vi "Test Report Contain Failiing TestCase Name.vi"(8 "error in (no error)":errorcluster, 11 "XML Report Test in":refnum<class "XML Report Test.lvclass">) -> (0 "error out":errorcluster, 3 "XML Report Test out":refnum<class "XML Report Test.lvclass">)   [LabVIEW 2020, in "XML Report Test.lvclass"]
uses:
  XML Report Test.lvclass
  source/Plugins/XML Report/XML Report.lvclass
  XML Report Test.lvclass/XML Report Test.ctl
  source/Core/Result/Result.ctl
  source/Core/Result/Status.ctl
  source/Core/Result/Type.ctl
  source/Core/Result/Result.lvlib
panel:
  out "Report Content":string
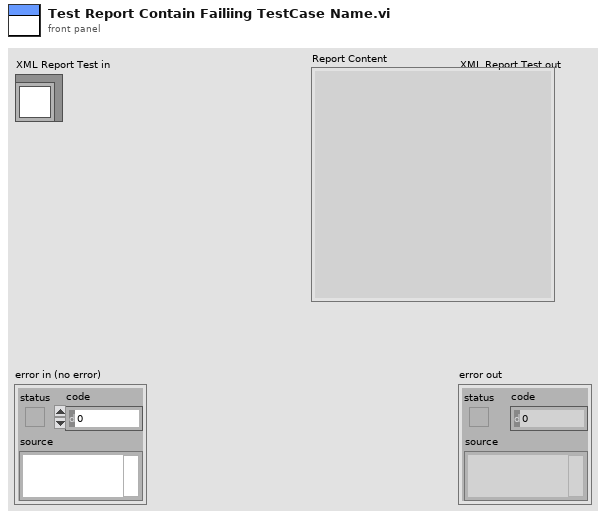
[diagram p1: front panel]
types:
  T1 = typedef "Result.lvlib/Result.ctl" = cluster{"Name":string, "Message":string, "Description":string, "Status":T2, "Result Type":T3, "Execution Time":dbl}
  T2 = typedef "Result.lvlib/Status.ctl" = enum16{"", "Passed", "Failed", "Error", "Skipped", "Setup Error", "Broken", "Teardown Error"}
  T3 = typedef "Result.lvlib/Type.ctl" = enum16{"Method", "Case", "Suite", "Pass", "Fail", "Skip", "Pass if", "Fail if", "Pass if Error", "Fail if Error", "Pass if Equal", "Fail if Equal"}
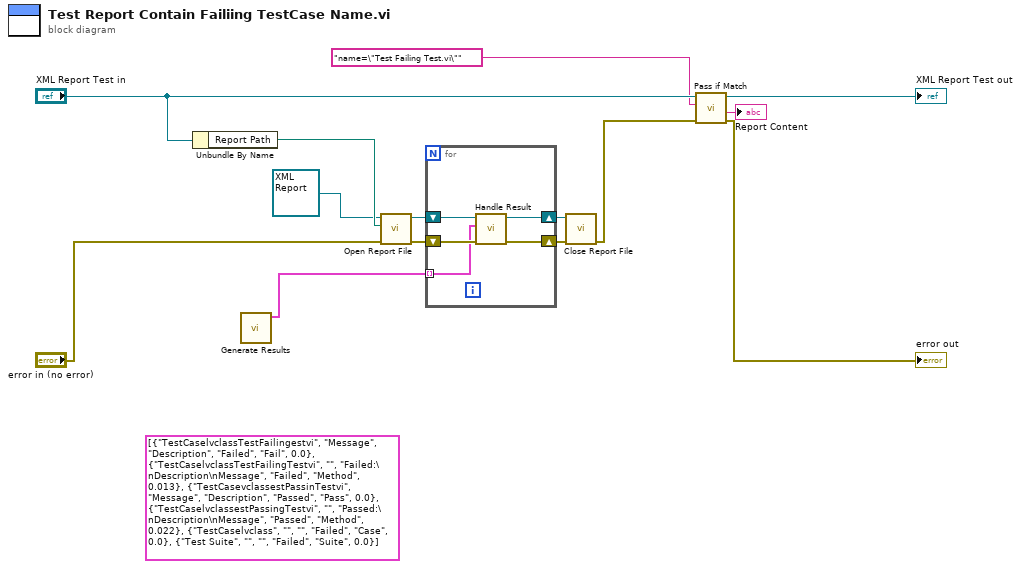
[diagram p0: block diagram]
diagram:
  (unwired) T1[] [{"Name"="TestCaselvclassTestFailingestvi", "Message"="Message", "Description"="Description", "Status"=enum."Failed", "Result Type"=enum."Fail", "Execution Time"=0.0}, {"Name"="TestCaselvclassTestFailingTestvi", "Message"="", "Description"="Failed:\nDescription\nMessage", "Status"=enum."Failed", "Result Type"=enum."Method", "Execution Time"=0.013}, {"Name"="TestCasevclassestPassinTestvi", "Message"="Message", "Description"="Description", "Status"=enum."Passed", "Result Type"=enum."Pass", "Execution Time"=0.0}, {"Name"="TestCaselvclassestPassingTestvi", "Message"="", "Description"="Passed:\nDescription\nMessage", "Status"=enum."Passed", "Result Type"=enum."Method", "Execution Time"=0.022}, {"Name"="TestCaselvclass", "Message"="", "Description"="", "Status"=enum."Failed", "Result Type"=enum."Case", "Execution Time"=0.0}, {"Name"="Test Suite", "Message"="", "Description"="", "Status"=enum."Failed", "Result Type"=enum."Suite", "Execution Time"=0.0}] ("Data")
  n1 = Unbundle By Name("XML Report Test in") -> ("Report Path"=w8:path)
  n2 = call "Generate Results.vi"() -> ("Data"=w1:T1[])  [unwired: 10 in, 1 out]
  n3 = call-dynamic "Open Report File.vi"("error in (no error)"="error in (no error)", "Report Path"=w8, "XML Report In"=refnum<class "XML Report.lvclass"> refnum) -> ("error out"=w14:errorcluster, "XML Report Out"=w4:refnum<class "XML Report.lvclass">)  [unwired: 7 in]
  n4 = for {
    shift-right: [w18] -> w5
    shift-left: w14 -> [w19]
    shift-right: [w16] -> w3
    shift-left: w4 -> [w17]
    tunnel: w1 -> [w15] mode=indexing
    n5 = call-dynamic "Handle Result.vi"("error in (no error)"=w19, "Result"=w15, "XML Report In"=w17) -> ("error out"=w18:errorcluster, "XML Report Out"=w16:refnum<class "XML Report.lvclass">)  [unwired: 7 in]
  }
  n6 = call-dynamic "Close Report File.vi"("error in (no error)"=w5, "XML Report In"=w3) -> ("error out"=w10:errorcluster)  [unwired: 9 in]
  n7 = call "Pass if Match.vi"("error in (no error)"=w10, "regular expression"="name=\"Test Failing Test.vi\"", "XML Report Test in"="XML Report Test in") -> ("error out"=→"error out":errorcluster, "Report Content"=→"Report Content":string, "XML Report Test out"=→"XML Report Test out":refnum<class "XML Report Test.lvclass">)  [unwired: 6 in]
